vi "Fetch Background Measurements (All).vi"(0 "VISA resource name":refnum<visa-resource-name>, 11 "error in (no error)":errorcluster) -> (4 "VISA resource name out":refnum<visa-resource-name>, 6 "Extended Measurements":T1, 15 "error out":errorcluster)   [LabVIEW 2020, in "NH Research Regenerative Test Series.lvlib"]
doc: "Returns the most recent measurements that are always being made by the hardware in the background (except while a waveform capture is being made)."
uses:
  NH Research Regenerative Test Series.lvlib
  Extended Background Measurements.ctl
  Background Measurements.ctl
  Peak Measurements.ctl
  Energy Measurements.ctl
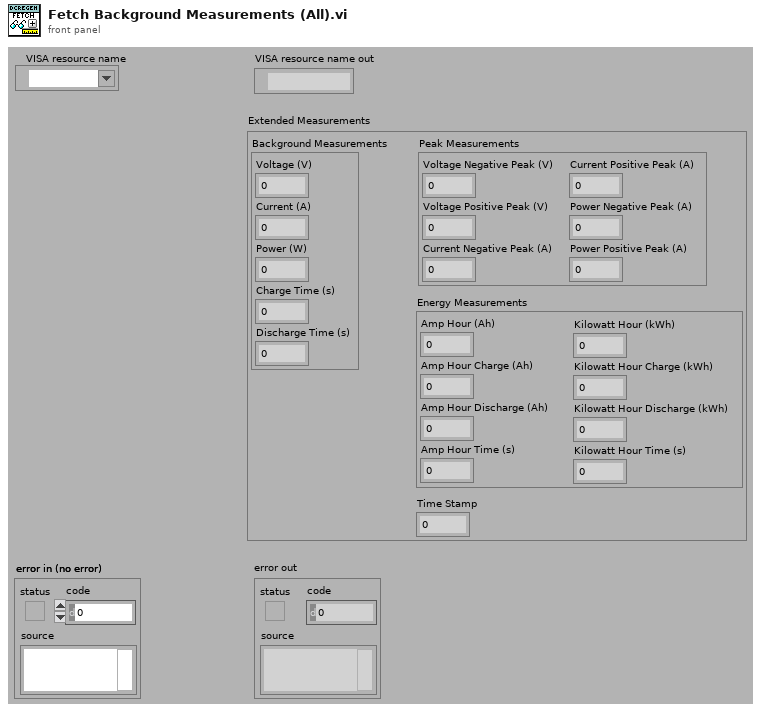
[diagram p1: front panel]
types:
  T1 = typedef "NH Research Regenerative Test Series.lvlib/Extended Background Measurements.ctl" = cluster{"Background Measurements":T2, "Peak Measurements":T3, "Energy Measurements":T4, "Time Stamp":dbl}
  T2 = typedef "NH Research Regenerative Test Series.lvlib/Background Measurements.ctl" = cluster{"Voltage (V)":dbl, "Current (A)":dbl, "Power (W)":dbl, "Charge Time (s)":dbl, "Discharge Time (s)":dbl}
  T3 = typedef "NH Research Regenerative Test Series.lvlib/Peak Measurements.ctl" = cluster{"Voltage Negative Peak (V)":dbl, "Voltage Positive Peak (V)":dbl, "Current Negative Peak (A)":dbl, "Current Positive Peak (A)":dbl, "Power Negative Peak (A)":dbl, "Power Positive Peak (A)":dbl}
  T4 = typedef "NH Research Regenerative Test Series.lvlib/Energy Measurements.ctl" = cluster{"Amp Hour (Ah)":dbl, "Amp Hour Charge (Ah)":dbl, "Amp Hour Discharge (Ah)":dbl, "Amp Hour Time (s)":dbl, "Kilowatt Hour (kWh)":dbl, "Kilowatt Hour Charge (kWh)":dbl, "Kilowatt Hour Discharge (kWh)":dbl, "Kilowatt Hour Time (s)":dbl}
  T5 = cluster{"[0]":dbl, "[1]":dbl, "[2]":dbl, "[3]":dbl, "[4]":dbl}
  T6 = cluster{"[0]":dbl, "[1]":dbl, "[2]":dbl, "[3]":dbl, "[4]":dbl, "[5]":dbl}
  T7 = cluster{"[0]":dbl, "[1]":dbl, "[2]":dbl, "[3]":dbl, "[4]":dbl, "[5]":dbl, "[6]":dbl, "[7]":dbl}
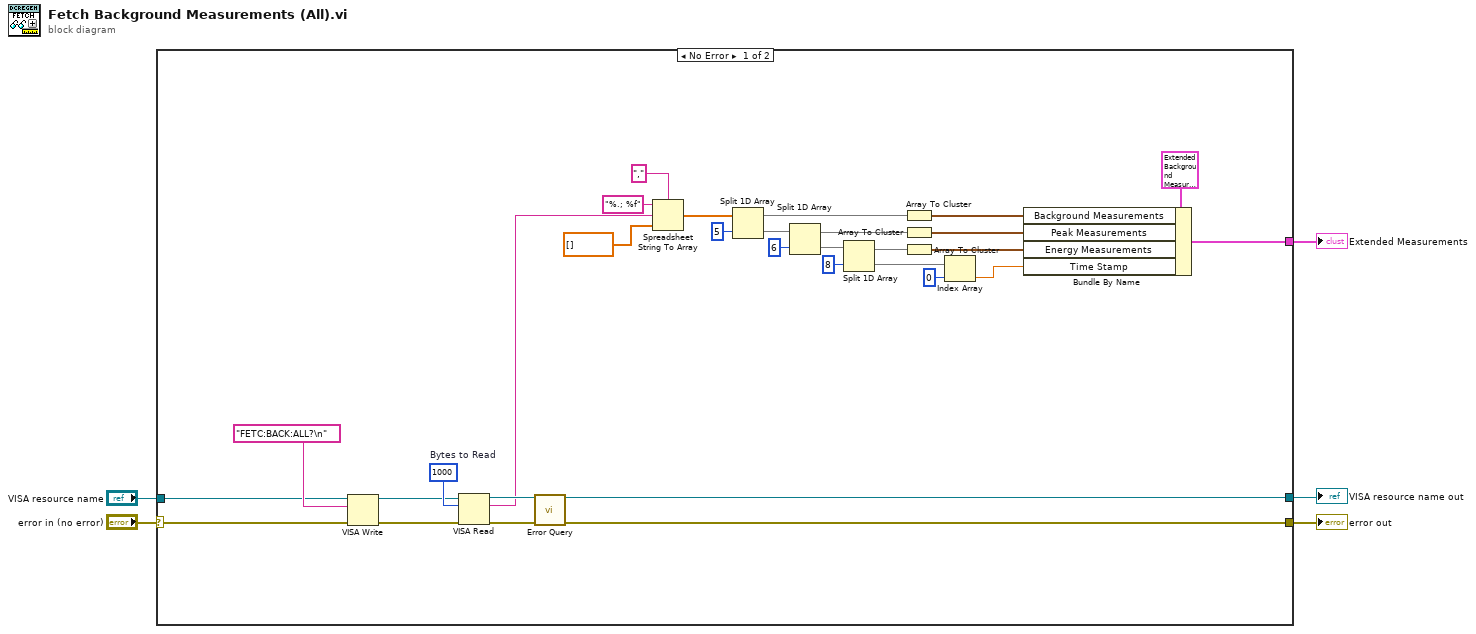
[diagram p0: block diagram]
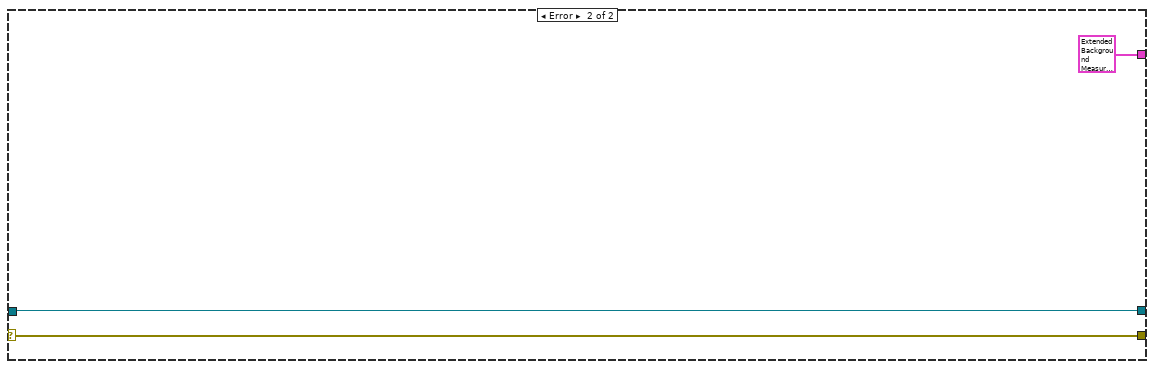
[diagram p2: hidden frame]
diagram:
  n1 = case shown="No Error" "error in (no error)" {
    selector: "error in (no error)" -> [w19 w39]
    tunnel: [w21 w39] -> w4
    tunnel: [w33 w38] -> w2
    tunnel: "VISA resource name" -> [w17 w38]
    tunnel: [w20 T1 {"Background Measurements"={"Voltage (V)"=nan, "Current (A)"=nan, "Power (W)"=nan, "Charge Time (s)"=nan, "Discharge Time (s)"=nan}, "Peak Measurements"={"Voltage Negative Peak (V)"=nan, "Voltage Positive Peak (V)"=nan, "Current Negative Peak (A)"=nan, "Current Positive Peak (A)"=nan, "Power Negative Peak (A)"=nan, "Power Positive Peak (A)"=nan}, "Energy Measurements"={"Amp Hour (Ah)"=nan, "Amp Hour Charge (Ah)"=nan, "Amp Hour Discharge (Ah)"=nan, "Amp Hour Time (s)"=nan, "Kilowatt Hour (kWh)"=nan, "Kilowatt Hour Charge (kWh)"=nan, "Kilowatt Hour Discharge (kWh)"=nan, "Kilowatt Hour Time (s)"=nan}, "Time Stamp"=nan}] -> w1
    frame No Error {
      w36 = u32 1000  # Bytes to Read
      n2 = VISA Write(VISA resource name=w17, write buffer="FETC:BACK:ALL?\n" ("Command"), error in (no error)=w19) -> (VISA resource name out=w34:refnum<visa-resource-name>, error out=w35:errorcluster)  [unwired: 1 out]
      n3 = VISA Read(VISA resource name=w34, byte count=w36, error in (no error)=w35) -> (VISA resource name out=w32:refnum<visa-resource-name>, read buffer=w27:string, error out=w31:errorcluster)  [unwired: 1 out]
      n4 = call "Error Query.vi"("VISA resource name"=w32, "error in (no error)"=w31) -> ("VISA resource name out"=w33:refnum<visa-resource-name>, "error out"=w21:errorcluster)  [unwired: 10 in, 2 out]
      n5 = Spreadsheet String To Array(delimiter (Tab)=",", format string="%.; %f", spreadsheet string=w27, array type (2D Dbl)=dbl[] []) -> (array=w25:dbl[])
      n6 = Split 1D Array(array=w25, index=5) -> (first subarray=w23:dbl[], second subarray=w16:dbl[])
      n7 = Split 1D Array(array=w16, index=6) -> (first subarray=w14:dbl[], second subarray=w12:dbl[])
      n8 = Split 1D Array(array=w12, index=8) -> (first subarray=w10:dbl[], second subarray=w9:dbl[])
      n9 = Array To Cluster(array=w23) -> (cluster=w22:T5)
      n10 = Array To Cluster(array=w14) -> (cluster=w13:T6)
      n11 = Array To Cluster(array=w10) -> (cluster=w6:T7)
      n12 = Index Array(array=w9, index=0) -> (element=w7:dbl)
      n13 = Bundle By Name(cluster=T1 {"Background Measurements"={"Voltage (V)"=0.0, "Current (A)"=0.0, "Power (W)"=0.0, "Charge Time (s)"=0.0, "Discharge Time (s)"=0.0}, "Peak Measurements"={"Voltage Negative Peak (V)"=0.0, "Voltage Positive Peak (V)"=0.0, "Current Negative Peak (A)"=0.0, "Current Positive Peak (A)"=0.0, "Power Negative Peak (A)"=0.0, "Power Positive Peak (A)"=0.0}, "Energy Measurements"={"Amp Hour (Ah)"=0.0, "Amp Hour Charge (Ah)"=0.0, "Amp Hour Discharge (Ah)"=0.0, "Amp Hour Time (s)"=0.0, "Kilowatt Hour (kWh)"=0.0, "Kilowatt Hour Charge (kWh)"=0.0, "Kilowatt Hour Discharge (kWh)"=0.0, "Kilowatt Hour Time (s)"=0.0}, "Time Stamp"=0.0} ("Extended Measurements"), "Background Measurements"=w22, "Peak Measurements"=w13, "Energy Measurements"=w6, "Time Stamp"=w7) -> (w20:T1)
    }
    frame Error {
    }
  }
  "error out" <- w4
  "VISA resource name out" <- w2
  "Extended Measurements" <- w1
